vi "UsrProfiles-Source-Default user profile name.vi"() -> (3 "Default user's profile file name & extension":string)   [LabVIEW 2017]
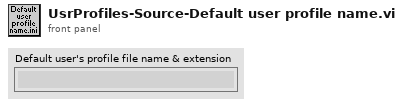
[diagram p1: front panel]
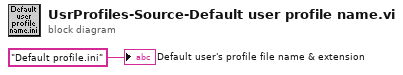
[diagram p0: block diagram]
diagram:
  "Default user's profile file name & extension" <- "Default profile.ini" ("y")
